vi "SFC_Split Combination.vi"(6 "UserNo":string, 7 "ProdLine":string, 8 "error in (no error)":errorcluster caption="错误输入（无错误）", 9 "Process":string, 10 "ParentSN":string, 11 "Traceability 引用句柄":refnum<k24>) -> (0 "error out":errorcluster caption="错误输出", 2 "SFC_SplitCombination":string, 3 "Traceability 引用句柄输出":refnum<k24>)   [LabVIEW 2014, in "Traceability.lvlib"]
uses:
  D:/webservice/Traceability.dll
  Traceability.dll
  Traceability.lvlib
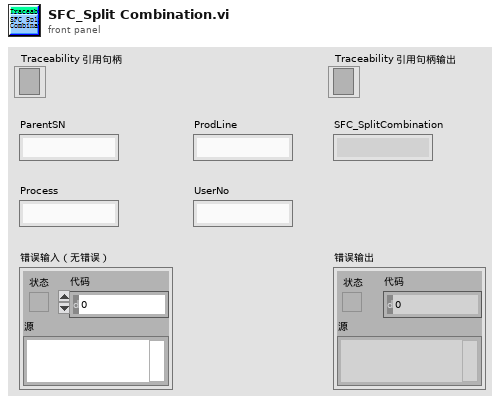
[diagram p1: front panel]
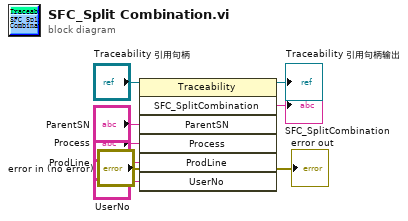
[diagram p0: block diagram]
diagram:
  n1 = invoke class="Traceability" method="SFC_SplitCombination"(reference="Traceability 引用句柄", error in="error in (no error)", "ParentSN"="ParentSN", "Process"="Process", "ProdLine"="ProdLine", "UserNo"="UserNo") -> (reference out=→"Traceability 引用句柄输出":refnum<k24>, error out=→"error out":errorcluster, "SFC_SplitCombination"=→"SFC_SplitCombination":string)  [unwired: 1 in, 4 out]
